vi "Write.vi"(8 "Error In":errorcluster, 10 "Cluster":variant, 11 "Path":path) -> (0 "Error Out":errorcluster)   [LabVIEW 2016, in "Configit.lvlib"]
doc: "Writes a named cluster to file in a human readable format that can be read back in using Configit Read."
uses:
  Configit.lvlib
  Insert Error.vi
  GetTypeInfo.vi
  <vilib>/Waveform/DWDTOps.llb/DWDT Empty Digital.vi
  <vilib>/Waveform/DTblOps.llb/DTbl Empty Digital.vi
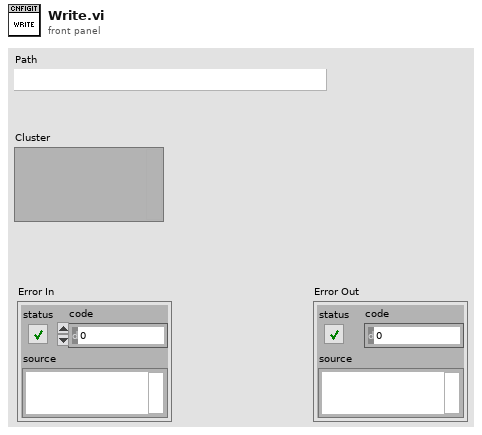
[diagram p1: front panel]
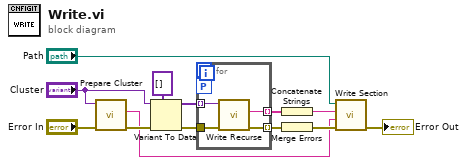
[diagram p0: block diagram]
diagram:
  n1 = call "Prepare Cluster.vi"("Error In"="Error In", "Default Cluster"="Cluster") -> ("Error Out"=w11:errorcluster, "Name"=w2:string)  [unwired: 8 in]
  n2 = Variant To Data(error in=w11, type=variant[] [], Variant="Cluster") -> (data=w9:variant[], error out=w8:errorcluster)
  n3 = for {
    tunnel: w9 -> [w17] mode=indexing
    tunnel: w8 -> [w16]
    tunnel: [w15] -> w7 mode=indexing
    tunnel: [w14] -> w6 mode=indexing
    workers-P: _ -> [_]
    n4 = call "Write Recurse.vi"("Error In"=w16, "Variant"=w17) -> ("Error Out"=w14:errorcluster, "String"=w15:string)  [unwired: 8 in]
  }
  n5 = Concatenate Strings(w7) -> (w4:string)
  n6 = Merge Errors(w6) -> (w5:errorcluster)
  n7 = call "Write Section.vi"("Error In"=w5, "Section"=w2, "Data"=w4, "Path"="Path") -> ("Error Out"=→"Error Out":errorcluster)  [unwired: 7 in]
